vi "Set MCP Gating.vi"(8 "error in (no error)":errorcluster, 11 "gating":i32) -> (0 "error out":errorcluster, 3 "function return":u32)   [LabVIEW 2014, in "atmcd32d.lvlib"]
doc: "unsigned int WINAPI SetMCPGating(int gating);"
uses:
  atmcd32d.lvlib
  atmcd32d.dll
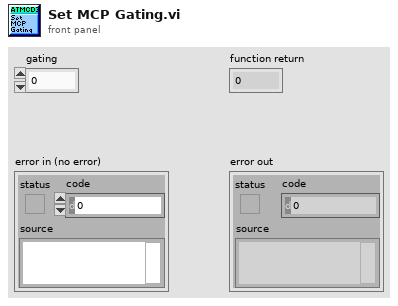
[diagram p1: front panel]
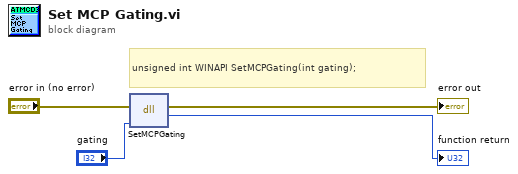
[diagram p0: block diagram]
diagram:
  # "unsigned int WINAPI SetMCPGating(int gating);"
  n1 = dll-call lib="C:/Users/Bakir/Documents/Lambda2-Testing/lib/Andorlib/atmcd32d.*" fn="SetMCPGating"(error in="error in (no error)", "gating"="gating") -> (error out=→"error out":errorcluster, →"function return":u32)  [unwired: 3 in, 1 out]
